vi "lvssh2_session_callback_receive_handler_64.vi"(9 "lvssh2_session_callback_receive":refnum<vi>, 10 "Stop Event Ref":refnum<user-event>, 11 "User Event Ref":refnum<user-event>) -> ()   [LabVIEW 2017, in "libssh2.lvlib"]
uses:
  libssh2.lvlib
  lvssh2_session_callback_receive_function_input_args_64.ctl
  lvssh2_extensions_64.dll
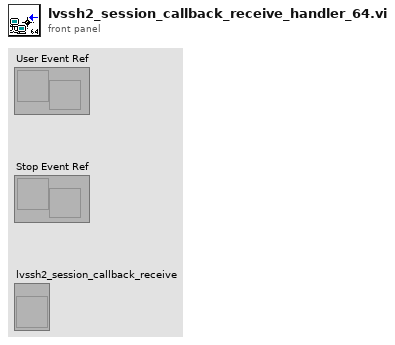
[diagram p1: front panel]
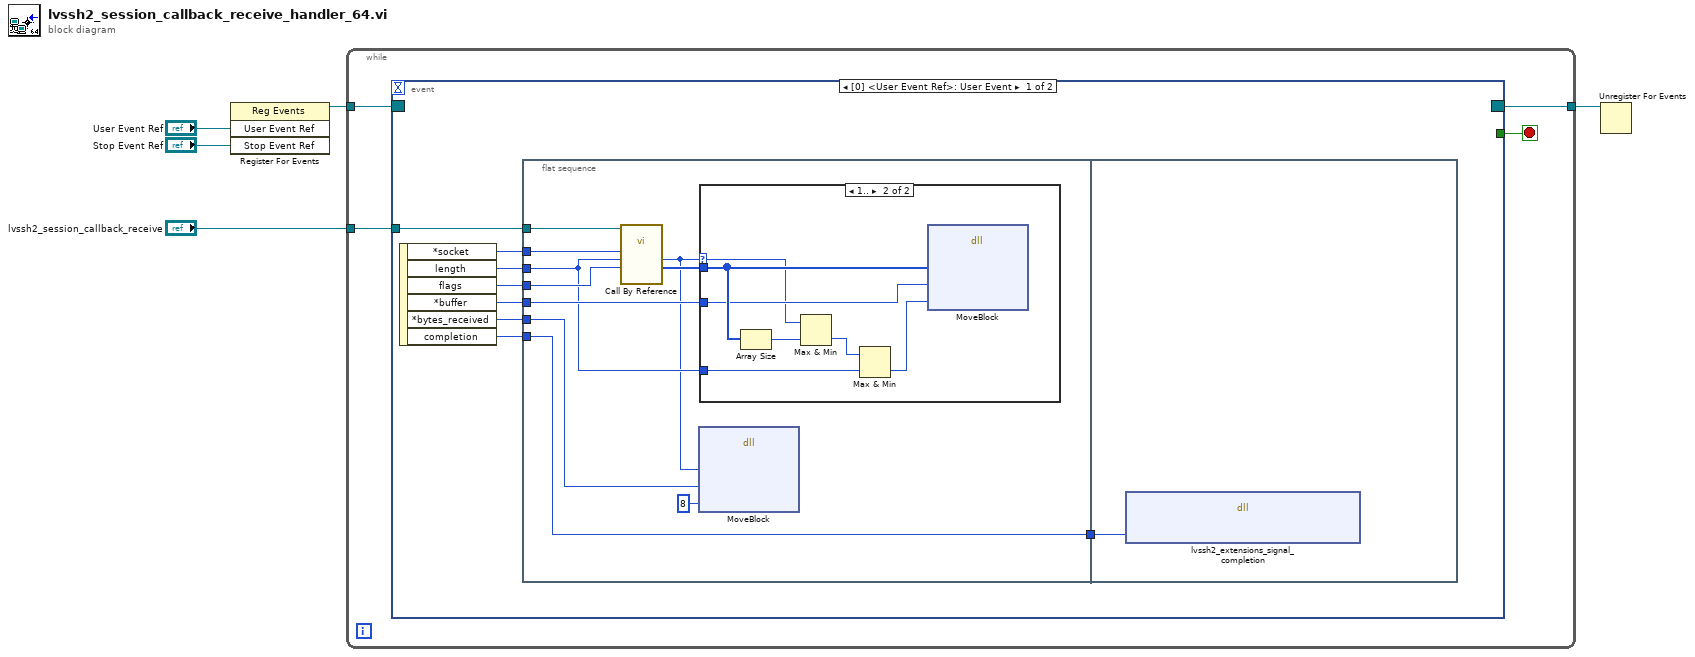
[diagram p0: block diagram]
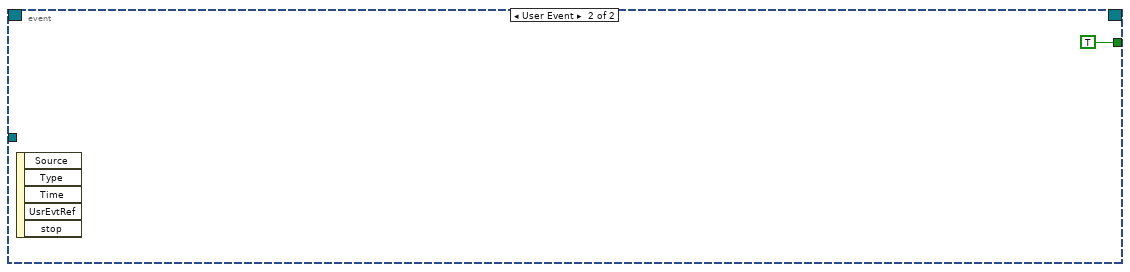
[diagram p3: hidden frame]
diagram:
  n1 = register-events("User Event Ref", "Stop Event Ref") -> (reference out=w4:refnum<event-registration>)  [unwired: 2 in, 1 out]
  n2 = while {
    tunnel: "lvssh2_session_callback_receive" -> [w9]
    tunnel: w4 -> [w8]
    tunnel: [w7] -> w1
    stop <- w6 stop-if-true
    n3 = event shown="[0] <User Event Ref>: User Event" {
      selector: w8 -> [_ _]
      dyn-events: [_ _] -> w7
      timeout: _ -> [_ _]
      tunnel: w9 -> [w16 _]
      tunnel: [_ TRUE] -> w6
      event User Event {
        n4 = event-data() -> ("*socket"=w15:u64, "length"=w14:u64, "flags"=w13:i32, "*buffer"=w12:u64, "*bytes_received"=w11:u64, "completion"=w10:u64)  [unwired: 1 in]
        n5 = flat-sequence {
          tunnel: w16 -> [w27]
          tunnel: w15 -> [w26]
          tunnel: w13 -> [w25]
          tunnel: w12 -> [w23]
          tunnel: w14 -> [w22]
          tunnel: w11 -> [w20]
          tunnel: [w18] -> w17
          tunnel: w10 -> [w18]
          tunnel: w17 -> [w35]
          frame #0 {
            n6 = call-by-ref "?"(reference=w27, "flags"=w25, "length"=w22, "socket"=w26) -> ("buffer"=w24:u8[], "bytes received"=w21:i64)  [unwired: 7 in, 3 out]
            n7 = dll-call lib="LabVIEW" fn="MoveBlock"("ps"=w21, "pd"=w20, "size"=u64 8) -> ()  [unwired: 7 in, 2 out]
            n8 = case shown="1.." w21 {
              selector: w21 -> [_ w31]
              tunnel: w24 -> [_ w34]
              tunnel: w23 -> [_ w33]
              tunnel: w22 -> [_ w30]
              frame Default {
              }
              frame 1.. {
                n9 = Array Size(array=w34) -> (size(s)=w32:i32)
                n10 = Max & Min(x=w31, y=w32) -> (min(x,y)=w29:i64)  [unwired: 1 out]
                n11 = Max & Min(x=w29, y=w30) -> (min(x,y)=w28:u64)  [unwired: 1 out]
                n12 = dll-call lib="LabVIEW" fn="MoveBlock"("ps"=w34, "pd"=w33, "size"=w28) -> ()  [unwired: 7 in, 2 out]
              }
            }
          }
          frame #1 {
            n13 = dll-call lib="C:/Users/Pascal/Projects/Home/lvssh2/libssh2/lvssh2_extensions**.*" fn="lvssh2_extensions_signal_completion"("completion"=w35) -> ()  [unwired: 5 in, 2 out]
          }
        }
      }
      event User Event {
        n14 = event-data() -> ()  [unwired: 1 in, 5 out]
      }
    }
  }
  n15 = Unregister For Events(event registration refnum=w1) -> ()  [unwired: 1 in, 1 out]
